vi "FGV Betriebsdaten.vi"(6 "Aktionen":T11, 8 "Parameter Sensoren":sgl[](array[numeric]), 9 "Sonstige":sgl[](array[numeric]), 10 "PID-Parameter":sgl[][](array[numeric]), 11 "Anlagen-Grenzwerte":sgl[][](array[numeric])) -> (0 "Parameter Sensoren":T1 {"Druck Kalter Block" format="%#_5g"; "Offset Druck FTIR IAG" format="%#_5g"; "Offset Druck CG" format="%#_5g"; "Offset Druck CG PMA" format="%#_5g"; "Offset Durchfl.PMA" format="%#_5g"; "Offset Druck Umgebung" format="%#_5g"; "Offset Druck Ausgang" format="%#_5g"; "Offset Durchfl.FTIR" format="%#_5g"; "Kal.Durchfl.PMA" format="%.3g"; "Kal.Durchfl.FTIR" format="%.3g"}, 1 "Sonstige":T2 {"ext. Befüllung" items=["Deaktiviert", "Aktiviert"]; "Dichtheitstest Umfang" items=["Pumpe / Filter / FT-IR / PNS", "Pumpe / Filter / FT-IR", "Filter / FT-IR", "FT-IR"]; "Befüllung aktiv" items=["Deaktiviert", "Aktiviert"]}, 2 "PID-Parameter":T6 {"Heizung\nFB-Druckregler"."max. OUT" format="%#_5g"; "Heizung\nFB-Druckregler"."Regelzonengr." format="%#_5g"; "Heizung\nFB-Druckregler"."D-Anteil" format="%#_5g"; "Heizung\nFB-Druckregler"."I-Anteil" format="%#_5g"; "Heizung\nFB-Druckregler"."P-Anteil" format="%.1f"; "Heizleitung\nExtern"."max. OUT" format="%#_5g"; "Heizleitung\nExtern"."Regelzonengr." format="%#_5g"; "Heizleitung\nExtern"."D-Anteil" format="%#_5g"; "Heizleitung\nExtern"."I-Anteil" format="%#_5g"; "Heizleitung\nExtern"."P-Anteil" format="%.1f"; "Heizung\nHeizleitungen"."max. OUT" format="%#_5g"; "Heizung\nHeizleitungen"."Regelzonengr." format="%#_5g"; "Heizung\nHeizleitungen"."D-Anteil" format="%#_5g"; "Heizung\nHeizleitungen"."I-Anteil" format="%#_5g"; "Heizung\nHeizleitungen"."P-Anteil" format="%.1f"; "Heizung\nPumpe"."max. OUT" format="%#_5g"; "Heizung\nPumpe"."Regelzonengr." format="%#_5g"; "Heizung\nPumpe"."D-Anteil" format="%#_5g"; "Heizung\nPumpe"."I-Anteil" format="%#_5g"; "Heizung\nPumpe"."P-Anteil" format="%.1f"; "Heizung\nFilterblock"."max. OUT" format="%#_5g"; "Heizung\nFilterblock"."Regelzonengr." format="%#_5g"; "Heizung\nFilterblock"."D-Anteil" format="%#_5g"; "Heizung\nFilterblock"."I-Anteil" format="%#_5g"; "Heizung\nFilterblock"."P-Anteil" format="%.1f"}, 3 "Anlagen-Grenzwerte":T9 {"Heizleitung zu FT-IR:"."Abschalt-Max" format="%#_5g"; "Heizleitung zu FT-IR:"."Abschalt-Min" format="%#_5g"; "Heizleitung zu FT-IR:"."Warn-Max" format="%#_5g"; "Heizleitung zu FT-IR:"."Warn-Min" format="%#_5g"; "Heizleitung zu FT-IR:"."Sollwert" format="%#_5g"; "Heizleitung zu FT-IR:"."Regler" items=["inaktiv", "aktiv"]; "Druck Kalter Block:"."Abschalt-Max" format="%#_5g"; "Druck Kalter Block:"."Abschalt-Min" format="%#_5g"; "Druck Kalter Block:"."Warn-Max" format="%#_5g"; "Druck Kalter Block:"."Warn-Min" format="%#_5g"; "Druck Kalter Block:"."Sollwert" format="%#_5g"; "Druck Kalter Block:"."Regler" items=["inaktiv", "aktiv"]; "Durchfluss CalGas:"."Abschalt-Max" format="%#_5g"; "Durchfluss CalGas:"."Abschalt-Min" format="%#_5g"; "Durchfluss CalGas:"."Warn-Max" format="%#_5g"; "Durchfluss CalGas:"."Warn-Min" format="%#_5g"; "Durchfluss CalGas:"."Sollwert" format="%#_5g"; "Durchfluss CalGas:"."Regler" items=["inaktiv", "aktiv"]; "Heizleitung Extern SP2:"."Abschalt-Max" format="%#_5g"; "Heizleitung Extern SP2:"."Abschalt-Min" format="%#_5g"; "Heizleitung Extern SP2:"."Warn-Max" format="%#_5g"; "Heizleitung Extern SP2:"."Warn-Min" format="%#_5g"; "Heizleitung Extern SP2:"."Sollwert" format="%#_5g"; "Heizleitung Extern SP2:"."Regler" items=["inaktiv", "aktiv"]; "Gaskühler:"."Abschalt-Max" format="%#_5g"; "Gaskühler:"."Abschalt-Min" format="%#_5g"; "Gaskühler:"."Warn-Max" format="%#_5g"; "Gaskühler:"."Warn-Min" format="%#_5g"; "Gaskühler:"."Sollwert" format="%#_5g"; "Gaskühler:"."Regler" items=["inaktiv", "aktiv"]; "Heizleitung Extern SP1:"."Abschalt-Max" format="%#_5g"; "Heizleitung Extern SP1:"."Abschalt-Min" format="%#_5g"; "Heizleitung Extern SP1:"."Warn-Max" format="%#_5g"; "Heizleitung Extern SP1:"."Warn-Min" format="%#_5g"; "Heizleitung Extern SP1:"."Sollwert" format="%#_5g"; "Heizleitung Extern SP1:"."Regler" items=["inaktiv", "aktiv"]; "Schaltschranktemperatur:"."Abschalt-Max" format="%#_5g"; "Schaltschranktemperatur:"."Abschalt-Min" format="%#_5g"; "Schaltschranktemperatur:"."Warn-Max" format="%#_5g"; "Schaltschranktemperatur:"."Warn-Min" format="%#_5g"; "Schaltschranktemperatur:"."Sollwert" format="%#_5g"; "Schaltschranktemperatur:"."Regler" items=["inaktiv", "aktiv"]; "FT-IR Heizung Messzelle:"."Abschalt-Max" format="%#_5g"; "FT-IR Heizung Messzelle:"."Abschalt-Min" format="%#_5g"; "FT-IR Heizung Messzelle:"."Warn-Max" format="%#_5g"; "FT-IR Heizung Messzelle:"."Warn-Min" format="%#_5g"; "FT-IR Heizung Messzelle:"."Sollwert" format="%#_5g"; "FT-IR Heizung Messzelle:"."Regler" items=["inaktiv", "aktiv"]; "Heizung Pumpe:"."Abschalt-Max" format="%#_5g"; "Heizung Pumpe:"."Abschalt-Min" format="%#_5g"; "Heizung Pumpe:"."Warn-Max" format="%#_5g"; "Heizung Pumpe:"."Warn-Min" format="%#_5g"; "Heizung Pumpe:"."Sollwert" format="%#_5g"; "Heizung Pumpe:"."Regler" items=["inaktiv", "aktiv"]; "Heizung Filterblock:"."Abschalt-Max" format="%#_5g"; "Heizung Filterblock:"."Abschalt-Min" format="%#_5g"; "Heizung Filterblock:"."Warn-Max" format="%#_5g"; "Heizung Filterblock:"."Warn-Min" format="%#_5g"; "Heizung Filterblock:"."Sollwert" format="%#_5g"; "Heizung Filterblock:"."Regler" items=["inaktiv", "aktiv"]; "Heizleitungen intern:"."Abschalt-Max" format="%#_5g"; "Heizleitungen intern:"."Abschalt-Min" format="%#_5g"; "Heizleitungen intern:"."Warn-Max" format="%#_5g"; "Heizleitungen intern:"."Warn-Min" format="%#_5g"; "Heizleitungen intern:"."Sollwert" format="%#_5g"; "Heizleitungen intern:"."Regler" items=["inaktiv", "aktiv"]; "Druck Ausgang:"."Abschalt-Max" format="%#_5g"; "Druck Ausgang:"."Abschalt-Min" format="%#_5g"; "Druck Ausgang:"."Warn-Max" format="%#_5g"; "Druck Ausgang:"."Warn-Min" format="%#_5g"; "Druck Ausgang:"."Sollwert" format="%#_5g"; "Druck Ausgang:"."Regler" items=["inaktiv", "aktiv"]; "Durchfluss FT-IR:"."Abschalt-Max" format="%#_5g"; "Durchfluss FT-IR:"."Abschalt-Min" format="%#_5g"; "Durchfluss FT-IR:"."Warn-Max" format="%#_5g"; "Durchfluss FT-IR:"."Warn-Min" format="%#_5g"; "Durchfluss FT-IR:"."Sollwert" format="%#_5g"; "Durchfluss FT-IR:"."Regler" items=["inaktiv", "aktiv"]; "Eingangsdruck FT-IR:"."Abschalt-Max" format="%#_5g"; "Eingangsdruck FT-IR:"."Abschalt-Min" format="%#_5g"; "Eingangsdruck FT-IR:"."Warn-Max" format="%#_5g"; "Eingangsdruck FT-IR:"."Warn-Min" format="%#_5g"; "Eingangsdruck FT-IR:"."Sollwert" format="%#_5g"; "Eingangsdruck FT-IR:"."Regler" items=["inaktiv", "aktiv"]})   [LabVIEW 2020, in "Konfig-Dateien.lvlib"]
uses:
  Konfig-Dateien.lvlib
  FGV Betriebsdaten Aktionen.ctl
  Seiten/Anlagengrenzwerte/Anlagen-Grenzwerte Anzeige.ctl
  Seiten/Anlagengrenzwerte/Anlagen-Parameter Anzeige.ctl
  Seiten/Erweiterte Konfig/PID-Parameter Anzeige.ctl
  Seiten/Erweiterte Konfig/PID-Parameter.ctl
  Visualisierungs Elemente/Zahlen-Eingabefeld.ctl
  Seiten/Erweiterte Konfig/Sonstige Parameter.ctl
  Visualisierungs Elemente/Auswahlfeld.ctl
  Seiten/Log Konfig/Auswahlfeld aktiviert-deaktiviert.ctl
  Seiten/Erweiterte Konfig/Dichtheitstest Umfang.ctl
  Seiten/Erweiterte Konfig/Parameter Sensoren.ctl
  Seiten/Anlagengrenzwerte/Anlagengrenzwerte.lvlib
  Seiten/Erweiterte Konfig/Erweiterte Konfig.lvlib
  Seiten/Log Konfig/LogKonfig.lvlib
panel:
  # "sec"
  # "sec"
  # "°C"
  # "%"
  # "sec"
  # "sec"
  # "°C"
  # "%"
  # "sec"
  # "sec"
  # "°C"
  # "%"
  # "sec"
  # "sec"
  # "°C"
  # "%"
  # "sec"
  # "sec"
  # "°C"
  # "%"
  # "°C"
  # "°C"
  # "°C"
  # "mbar"
  # "mbar"
  # "mbar"
  # "l/min"
  # "l/min"
  # "l/min"
  # "°C"
  # "°C"
  # "°C"
  # "°C"
  # "°C"
  # "°C"
  # "°C"
  # "°C"
  # "°C"
  # "°C"
  # "°C"
  # "°C"
  # "°C"
  # "°C"
  # "°C"
  # "°C"
  # "°C"
  # "°C"
  # "°C"
  # "°C"
  # "°C"
  # "°C"
  # "°C"
  # "°C"
  # "mbar"
  # "mbar"
  # "mbar"
  # "l/min"
  # "l/min"
  # "l/min"
  # "atm"
  # "atm"
  # "atm"
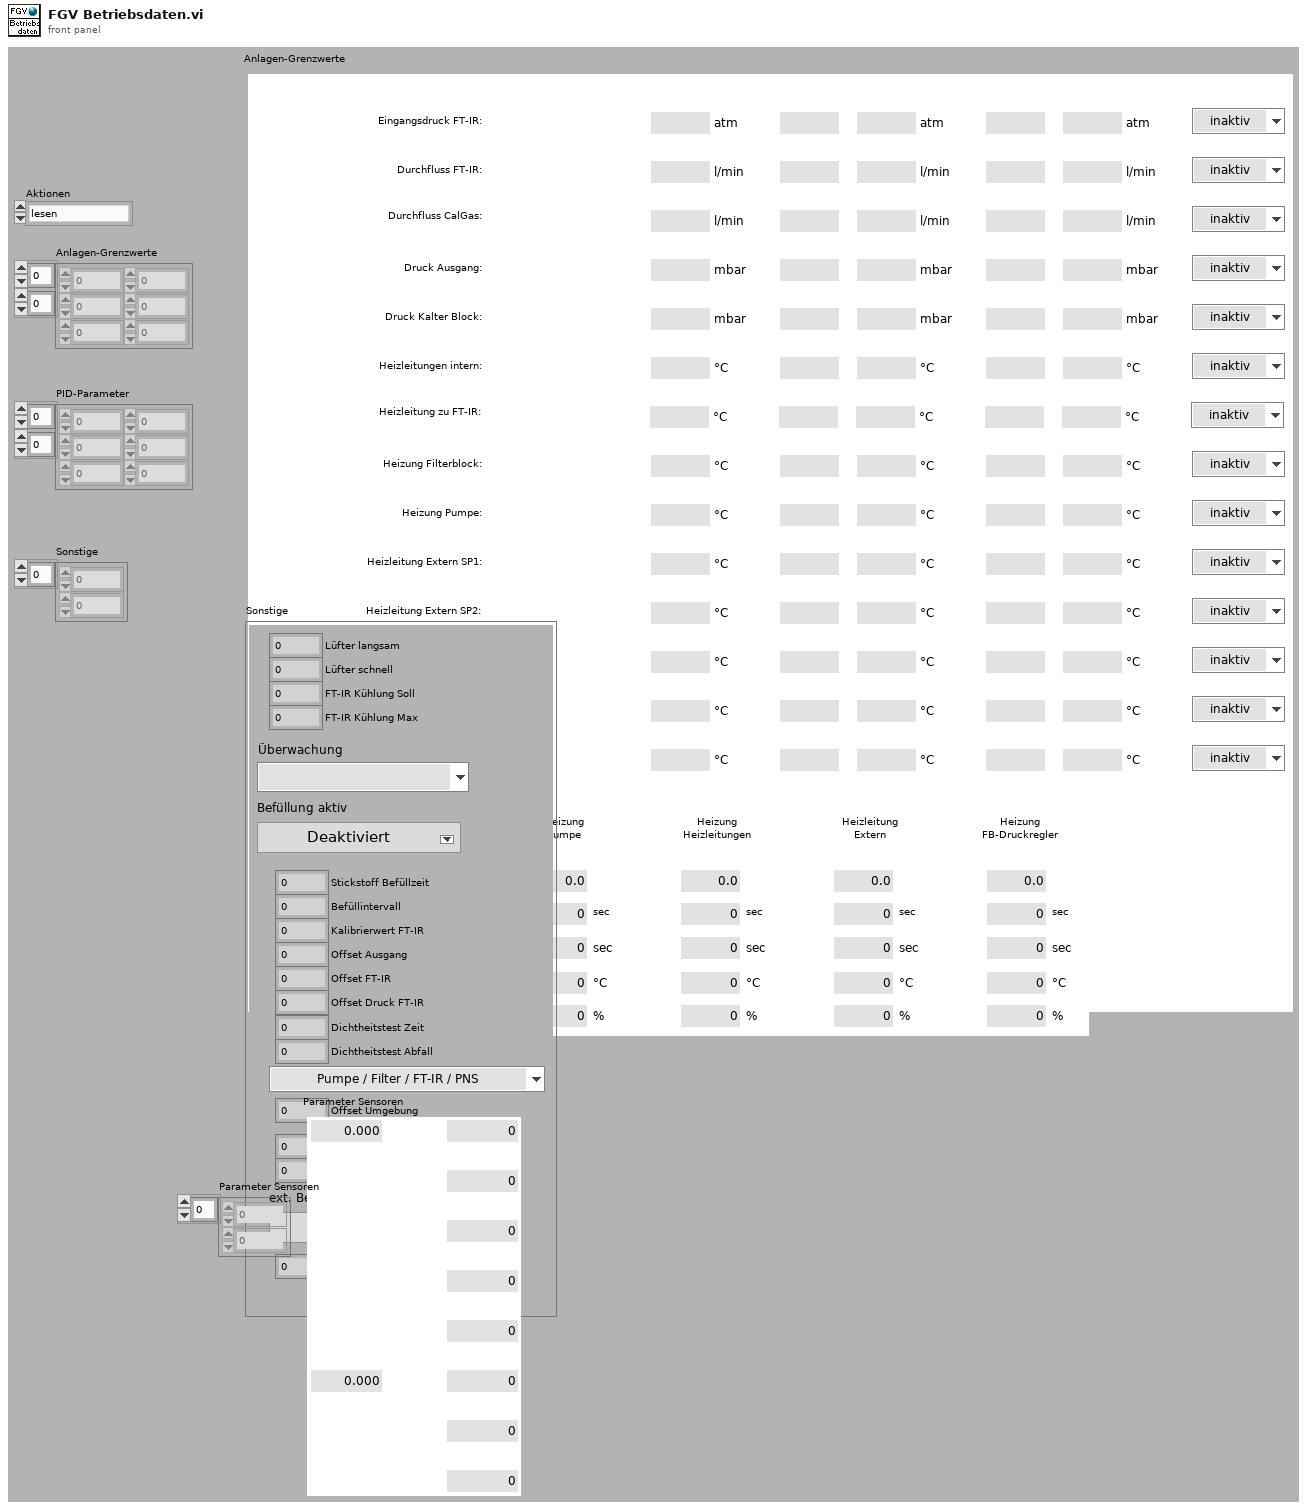
[diagram p1: front panel]
types:
  T1 = typedef "Erweiterte Konfig.lvlib/Parameter Sensoren.ctl" = cluster{"Kal.Durchfl.FTIR":sgl, "Kal.Durchfl.PMA":sgl, "Offset Durchfl.FTIR":sgl, "Offset Druck Ausgang":sgl, "Offset Druck Umgebung":sgl, "Offset Durchfl.PMA":sgl, "Offset Druck CG PMA":sgl, "Offset Druck CG":sgl, "Offset Druck FTIR IAG":sgl, "Druck Kalter Block":sgl}
  T2 = typedef "Erweiterte Konfig.lvlib/Sonstige Parameter.ctl" = cluster{"Lüfter langsam":sgl, "Lüfter schnell":sgl, "FT-IR Kühlung Soll":sgl, "FT-IR Kühlung Max":sgl, "Überwachung":T3, "Befüllung aktiv":T4, "Stickstoff Befüllzeit":sgl, "Befüllintervall":sgl, "Kalibrierwert FT-IR":sgl, "Offset Ausgang":sgl, "Offset FT-IR":sgl, "Offset Druck FT-IR":sgl, "Dichtheitstest Zeit":sgl, "Dichtheitstest Abfall":sgl, "Dichtheitstest Umfang":T5, "Offset Umgebung":sgl, "Max Taupunkt":sgl, "Pumpendrehzahl":sgl, "ext. Befüllung":T4, "Ext. Stickstoff Befüllzeit":sgl}
  T3 = typedef "Auswahlfeld.ctl" = u16
  T4 = typedef "LogKonfig.lvlib/Auswahlfeld aktiviert-deaktiviert.ctl" = u16
  T5 = typedef "Erweiterte Konfig.lvlib/Dichtheitstest Umfang.ctl" = u16
  T6 = typedef "Erweiterte Konfig.lvlib/PID-Parameter Anzeige.ctl" = cluster{"Heizung\nFilterblock":T7, "Heizung\nPumpe":T7, "Heizung\nHeizleitungen":T7, "Heizleitung\nExtern":T7, "Heizung\nFB-Druckregler":T7}
  T7 = typedef "Erweiterte Konfig.lvlib/PID-Parameter.ctl" = cluster{"P-Anteil":T8, "I-Anteil":T8, "D-Anteil":T8, "Regelzonengr.":T8, "max. OUT":T8}
  T8 = typedef "Zahlen-Eingabefeld.ctl" = sgl
  T9 = typedef "Anlagengrenzwerte.lvlib/Anlagen-Grenzwerte Anzeige.ctl" = cluster{"Eingangsdruck FT-IR:":T10, "Durchfluss FT-IR:":T10, "Durchfluss CalGas:":T10, "Druck Ausgang:":T10, "Druck Kalter Block:":T10, "Heizleitungen intern:":T10, "Heizleitung zu FT-IR:":T10, "Heizung Filterblock:":T10, "Heizung Pumpe:":T10, "Heizleitung Extern SP1:":T10, "Heizleitung Extern SP2:":T10, "FT-IR Heizung Messzelle:":T10, "Schaltschranktemperatur:":T10, "Gaskühler:":T10}
  T10 = typedef "Anlagengrenzwerte.lvlib/Anlagen-Parameter Anzeige.ctl" = cluster{"Sollwert":sgl, "Warn-Min":sgl, "Warn-Max":sgl, "Abschalt-Min":sgl, "Abschalt-Max":sgl, "Regler":u16}
  T11 = typedef "Konfig-Dateien.lvlib/FGV Betriebsdaten Aktionen.ctl" = enum16{"lesen", "Anlagengrenzw.", "PID Param.", "Sonstige", "Sensor Para."}
  T12 = cluster{"Parameter Sensoren[0]":sgl, "Parameter Sensoren[1]":sgl, "Parameter Sensoren[2]":sgl, "Parameter Sensoren[3]":sgl, "Parameter Sensoren[4]":sgl, "Parameter Sensoren[5]":sgl, "Parameter Sensoren[6]":sgl, "Parameter Sensoren[7]":sgl, "Parameter Sensoren[8]":sgl, "Parameter Sensoren[9]":sgl}
  T13 = cluster{"Anlagen-Grenzwerte[0]":sgl, "Anlagen-Grenzwerte[1]":sgl, "Anlagen-Grenzwerte[2]":sgl, "Anlagen-Grenzwerte[3]":sgl, "Anlagen-Grenzwerte[4]":sgl, "Anlagen-Grenzwerte[5]":sgl}
  T14 = cluster{"[0]":cluster{"Anlagen-Grenzwerte[0]":sgl, "Anlagen-Grenzwerte[1]":sgl, "Anlagen-Grenzwerte[2]":sgl, "Anlagen-Grenzwerte[3]":sgl, "Anlagen-Grenzwerte[4]":sgl, "Anlagen-Grenzwerte[5]":sgl}, "[1]":cluster{"Anlagen-Grenzwerte[0]":sgl, "Anlagen-Grenzwerte[1]":sgl, "Anlagen-Grenzwerte[2]":sgl, "Anlagen-Grenzwerte[3]":sgl, "Anlagen-Grenzwerte[4]":sgl, "Anlagen-Grenzwerte[5]":sgl}, "[2]":cluster{"Anlagen-Grenzwerte[0]":sgl, "Anlagen-Grenzwerte[1]":sgl, "Anlagen-Grenzwerte[2]":sgl, "Anlagen-Grenzwerte[3]":sgl, "Anlagen-Grenzwerte[4]":sgl, "Anlagen-Grenzwerte[5]":sgl}, "[3]":cluster{"Anlagen-Grenzwerte[0]":sgl, "Anlagen-Grenzwerte[1]":sgl, "Anlagen-Grenzwerte[2]":sgl, "Anlagen-Grenzwerte[3]":sgl, "Anlagen-Grenzwerte[4]":sgl, "Anlagen-Grenzwerte[5]":sgl}, "[4]":cluster{"Anlagen-Grenzwerte[0]":sgl, "Anlagen-Grenzwerte[1]":sgl, "Anlagen-Grenzwerte[2]":sgl, "Anlagen-Grenzwerte[3]":sgl, "Anlagen-Grenzwerte[4]":sgl, "Anlagen-Grenzwerte[5]":sgl}, "[5]":cluster{"Anlagen-Grenzwerte[0]":sgl, "Anlagen-Grenzwerte[1]":sgl, "Anlagen-Grenzwerte[2]":sgl, "Anlagen-Grenzwerte[3]":sgl, "Anlagen-Grenzwerte[4]":sgl, "Anlagen-Grenzwerte[5]":sgl}, "[6]":cluster{"Anlagen-Grenzwerte[0]":sgl, "Anlagen-Grenzwerte[1]":sgl, "Anlagen-Grenzwerte[2]":sgl, "Anlagen-Grenzwerte[3]":sgl, "Anlagen-Grenzwerte[4]":sgl, "Anlagen-Grenzwerte[5]":sgl}, "[7]":cluster{"Anlagen-Grenzwerte[0]":sgl, "Anlagen-Grenzwerte[1]":sgl, "Anlagen-Grenzwerte[2]":sgl, "Anlagen-Grenzwerte[3]":sgl, "Anlagen-Grenzwerte[4]":sgl, "Anlagen-Grenzwerte[5]":sgl}, "[8]":cluster{"Anlagen-Grenzwerte[0]":sgl, "Anlagen-Grenzwerte[1]":sgl, "Anlagen-Grenzwerte[2]":sgl, "Anlagen-Grenzwerte[3]":sgl, "Anlagen-Grenzwerte[4]":sgl, "Anlagen-Grenzwerte[5]":sgl}, "[9]":cluster{"Anlagen-Grenzwerte[0]":sgl, "Anlagen-Grenzwerte[1]":sgl, "Anlagen-Grenzwerte[2]":sgl, "Anlagen-Grenzwerte[3]":sgl, "Anlagen-Grenzwerte[4]":sgl, "Anlagen-Grenzwerte[5]":sgl}, "[10]":cluster{"Anlagen-Grenzwerte[0]":sgl, "Anlagen-Grenzwerte[1]":sgl, "Anlagen-Grenzwerte[2]":sgl, "Anlagen-Grenzwerte[3]":sgl, "Anlagen-Grenzwerte[4]":sgl, "Anlagen-Grenzwerte[5]":sgl}, "[11]":cluster{"Anlagen-Grenzwerte[0]":sgl, "Anlagen-Grenzwerte[1]":sgl, "Anlagen-Grenzwerte[2]":sgl, "Anlagen-Grenzwerte[3]":sgl, "Anlagen-Grenzwerte[4]":sgl, "Anlagen-Grenzwerte[5]":sgl}, "[12]":cluster{"Anlagen-Grenzwerte[0]":sgl, "Anlagen-Grenzwerte[1]":sgl, "Anlagen-Grenzwerte[2]":sgl, "Anlagen-Grenzwerte[3]":sgl, "Anlagen-Grenzwerte[4]":sgl, "Anlagen-Grenzwerte[5]":sgl}, "[13]":cluster{"Anlagen-Grenzwerte[0]":sgl, "Anlagen-Grenzwerte[1]":sgl, "Anlagen-Grenzwerte[2]":sgl, "Anlagen-Grenzwerte[3]":sgl, "Anlagen-Grenzwerte[4]":sgl, "Anlagen-Grenzwerte[5]":sgl}}
  T15 = cluster{"PID-Parameter[0]":sgl, "PID-Parameter[1]":sgl, "PID-Parameter[2]":sgl, "PID-Parameter[3]":sgl, "PID-Parameter[4]":sgl}
  T16 = cluster{"[0]":cluster{"PID-Parameter[0]":sgl, "PID-Parameter[1]":sgl, "PID-Parameter[2]":sgl, "PID-Parameter[3]":sgl, "PID-Parameter[4]":sgl}, "[1]":cluster{"PID-Parameter[0]":sgl, "PID-Parameter[1]":sgl, "PID-Parameter[2]":sgl, "PID-Parameter[3]":sgl, "PID-Parameter[4]":sgl}, "[2]":cluster{"PID-Parameter[0]":sgl, "PID-Parameter[1]":sgl, "PID-Parameter[2]":sgl, "PID-Parameter[3]":sgl, "PID-Parameter[4]":sgl}, "[3]":cluster{"PID-Parameter[0]":sgl, "PID-Parameter[1]":sgl, "PID-Parameter[2]":sgl, "PID-Parameter[3]":sgl, "PID-Parameter[4]":sgl}, "[4]":cluster{"PID-Parameter[0]":sgl, "PID-Parameter[1]":sgl, "PID-Parameter[2]":sgl, "PID-Parameter[3]":sgl, "PID-Parameter[4]":sgl}}
  T17 = cluster{"Sonstige[0]":sgl, "Sonstige[1]":sgl, "Sonstige[2]":sgl, "Sonstige[3]":sgl, "Sonstige[4]":sgl, "Sonstige[5]":sgl, "Sonstige[6]":sgl, "Sonstige[7]":sgl, "Sonstige[8]":sgl, "Sonstige[9]":sgl, "Sonstige[10]":sgl, "Sonstige[11]":sgl, "Sonstige[12]":sgl, "Sonstige[13]":sgl, "Sonstige[14]":sgl, "Sonstige[15]":sgl, "Sonstige[16]":sgl, "Sonstige[17]":sgl, "Sonstige[18]":sgl, "Sonstige[19]":sgl}
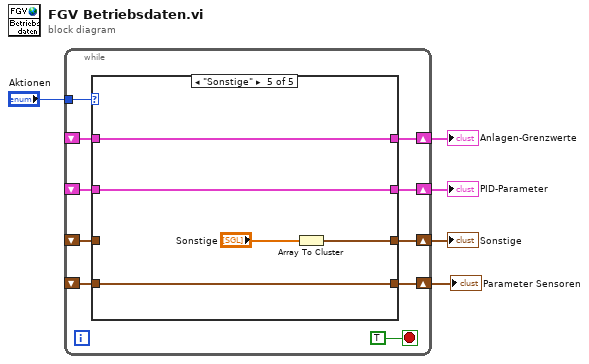
[diagram p0: block diagram]
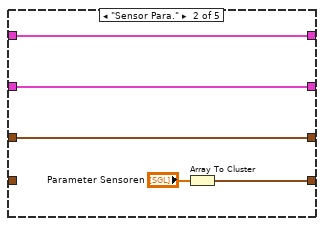
[diagram p3: hidden frame]
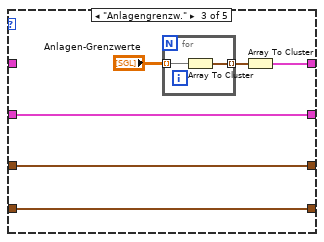
[diagram p4: hidden frame]
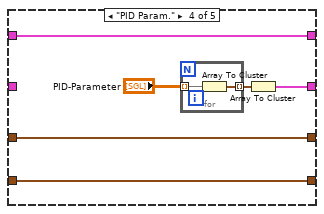
[diagram p5: hidden frame]
diagram:
  n1 = while {
    tunnel: "Aktionen" -> [w14]
    shift-right: [w12] -> w4
    shift-left: _ -> [w13]
    shift-right: [w10] -> w3
    shift-left: _ -> [w11]
    shift-right: [w8] -> w2
    shift-left: _ -> [w9]
    shift-right: [w7] -> w1
    shift-left: _ -> [w6]
    stop <- TRUE stop-if-true
    n2 = case shown="\"Sonstige\"" w14 {
      tunnel: w13 -> [w19 w24 _ w38 w45]
      tunnel: [w19 w24 w26 w38 w45] -> w12
      tunnel: w11 -> [w18 w23 w30 _ w44]
      tunnel: [w18 w23 w30 w34 w44] -> w10
      tunnel: w9 -> [w17 w22 w29 w37 _]
      tunnel: [w17 w22 w29 w37 w42] -> w8
      tunnel: [w16 w20 w25 w33 w41] -> w7
      tunnel: w6 -> [w16 _ w25 w33 w41]
      frame "lesen", Default {
      }
      frame "Sensor Para." {
        n3 = Array To Cluster(array="Parameter Sensoren") -> (cluster=w20:T12)
      }
      frame "Anlagengrenzw." {
        n4 = for {
          tunnel: "Anlagen-Grenzwerte" -> [w32] mode=indexing
          tunnel: [w31] -> w27 mode=indexing
          n5 = Array To Cluster(array=w32) -> (cluster=w31:T13)
        }
        n6 = Array To Cluster(array=w27) -> (cluster=w26:T14)
      }
      frame "PID Param." {
        n7 = for {
          tunnel: [w40] -> w36 mode=indexing
          tunnel: "PID-Parameter" -> [w39] mode=indexing
          n8 = Array To Cluster(array=w39) -> (cluster=w40:T15)
        }
        n9 = Array To Cluster(array=w36) -> (cluster=w34:T16)
      }
      frame "Sonstige" {
        n10 = Array To Cluster(array="Sonstige") -> (cluster=w42:T17)
      }
    }
  }
  "Anlagen-Grenzwerte" <- w4
  "PID-Parameter" <- w3
  "Sonstige" <- w2
  "Parameter Sensoren" <- w1
